vi "input.vi"(8 "error in":errorcluster, 10 "data table in":T1, 11 "dds runtime in":refnum<class "DDS runtime.lvclass">) -> (0 "error out":errorcluster, 2 "data table out":T1, 3 "dds runtime out":refnum<class "DDS runtime.lvclass">)   [LabVIEW 2013, in "DDS runtime.lvclass"]
doc: "Provides an interface for reading data from a module at runtime. While this interface performs no operations, a child should provide an override which may read from any open sessions, references, or interfaces."
uses:
  DDS runtime.lvclass
  <vilib>/NI/Tag Bus/table/data table.ctl
  DDS runtime.lvclass/DDS runtime.ctl
  <vilib>/NI/Tag Bus/table/data polymorphs/write one/write Double.vi
  <vilib>/NI/Tag Bus/table/data polymorphs/write one/write Single.vi
  <vilib>/NI/Tag Bus/table/data polymorphs/write one/write I64.vi
  <vilib>/NI/Tag Bus/table/data polymorphs/write one/write I32.vi
  <vilib>/NI/Tag Bus/table/data polymorphs/write one/write I16.vi
  <vilib>/NI/Tag Bus/table/data polymorphs/write one/write I8.vi
  <vilib>/NI/Tag Bus/table/data polymorphs/write one/write U64.vi
  <vilib>/NI/Tag Bus/table/data polymorphs/write one/write U32.vi
  <vilib>/NI/Tag Bus/table/data polymorphs/write one/write U16.vi
  <vilib>/NI/Tag Bus/table/data polymorphs/write one/write U8.vi
  <vilib>/NI/Tag Bus/table/data polymorphs/write one/write Boolean.vi
  <vilib>/NI/Tag Bus/table/data polymorphs/write one/write String.vi
  <vilib>/RTI DDS Toolkit for LabVIEW/VIs/Read_Num.vi
  <vilib>/RTI DDS Toolkit for LabVIEW/VIs/Read_NumSgl.vi
  <vilib>/RTI DDS Toolkit for LabVIEW/VIs/Read_NumI64.vi
  <vilib>/RTI DDS Toolkit for LabVIEW/VIs/Read_NumI32.vi
  <vilib>/RTI DDS Toolkit for LabVIEW/VIs/Read_NumI16.vi
  <vilib>/RTI DDS Toolkit for LabVIEW/VIs/Read_NumI8.vi
  <vilib>/RTI DDS Toolkit for LabVIEW/VIs/Read_NumU64.vi
  <vilib>/RTI DDS Toolkit for LabVIEW/VIs/Read_NumU32.vi
  <vilib>/RTI DDS Toolkit for LabVIEW/VIs/Read_NumU16.vi
  <vilib>/RTI DDS Toolkit for LabVIEW/VIs/Read_NumU8.vi
  <vilib>/RTI DDS Toolkit for LabVIEW/VIs/Read_Bool.vi
  <vilib>/RTI DDS Toolkit for LabVIEW/VIs/Read_String.vi
  <vilib>/NI/Tag Bus/table/data table.lvlib
  <vilib>/RTI DDS Toolkit for LabVIEW/Library/LVDDS_library.lvlib
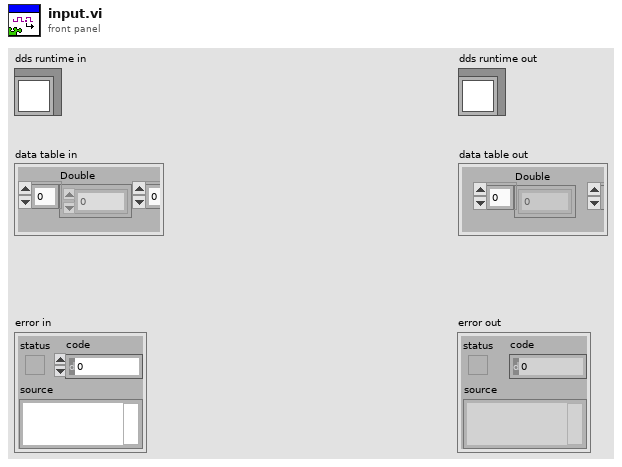
[diagram p1: front panel]
types:
  T1 = typedef "tag bus.lvlib/data table.lvlib/data table.ctl" = cluster{"Double":dbl[], "Single":sgl[], "I64":i64[], "I32":i32[], "I16":i16[], "I8":i8[], "U64":u64[], "U32":u32[], "U16":u16[], "U8":u8[], "Boolean":bool[], "String":string[], "Array of Double":cluster{"DBL Array":dbl[]}[], "Array of Single":cluster{"SGL Array":sgl[]}[], "Array of I64":cluster{"I64 Array":i64[]}[], "Array of I32":cluster{"I32 Array":i32[]}[], "Array of I16":cluster{"I16 Array":i16[]}[], "Array of I8":cluster{"I8 Array":i8[]}[], "Array of U64":cluster{"U64 Array":u64[]}[], "Array of U32":cluster{"U32 Array":u32[]}[], "Array of U16":cluster{"U16 Array":u16[]}[], "Array of U8":cluster{"U8 Array":u8[]}[], "Array of Boolean":cluster{"Boolean Array":bool[]}[], "Array of String":cluster{"String Array":string[]}[]}
  T2 = typedef "tag bus.lvlib/tag descriptor.lvclass/Data Type.ctl" = enum16{"Double", "Single", "I64", "I32", "I16", "I8", "U64", "U32", "U16", "U8", "Boolean", "String", "Array of Double", "Array of Single", "Array of I64", "Array of I32", "Array of I16", "Array of I8", "Array of U64", "Array of U32", "Array of U16", "Array of U8", "Array of Boolean", "Array of String"}
  T3 = cluster{"index":i32, "data type":T2, "ref num":u64, "new samples only":bool, "query condition":string}[]
  T4 = typedef "LVDDS_library.lvlib/DDS Sample Info.ctl" = cluster{"DDS_SampleStateKind":enum32{"DDS_INVALID_SAMPLE_STATE", "DDS_READ_SAMPLE_STATE", "DDS_NOT_READ_SAMPLE_STATE"}, "DDS_ViewStateKind":enum32{"DDS_INVALID_SAMPLE_STATE", "DDS_NEW_VIEW_STATE", "DDS_NOT_NEW_VIEW_STATE"}, "DDS_InstanceStateKind":enum32{"DDS_INVALID_STATE", "DDS_ALIVE_INSTANCE_STATE", "DDS_NOT_ALIVE_DISPOSED_INSTANCE_STATE", "", "DDS_NOT_ALIVE_NO_WRITERS_INSTANCE_STATE"}, "sec":i32, "nanosec":u32, "valid_data":bool}
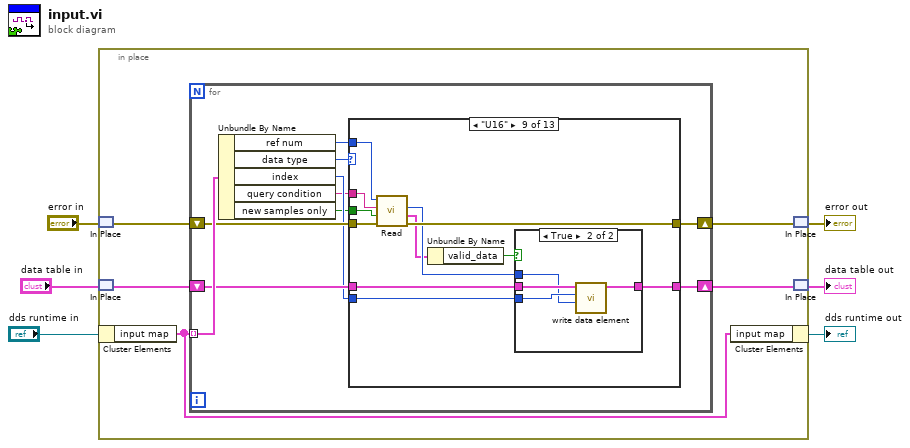
[diagram p0: block diagram]
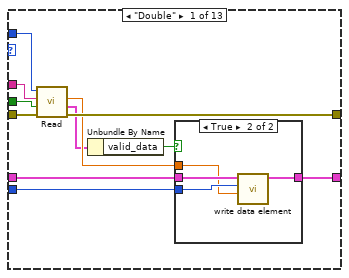
[diagram p2: hidden frame]
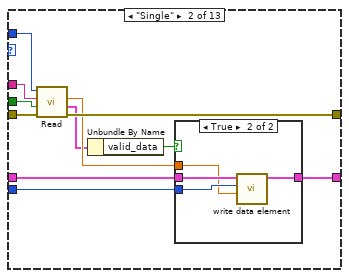
[diagram p4: hidden frame]
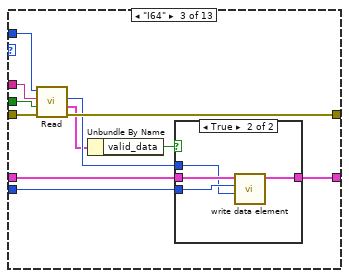
[diagram p6: hidden frame]
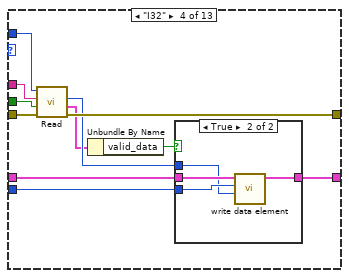
[diagram p8: hidden frame]
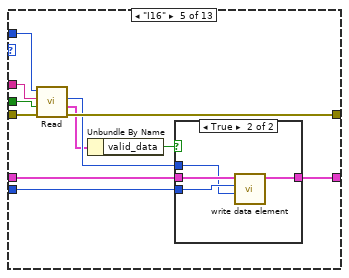
[diagram p10: hidden frame]
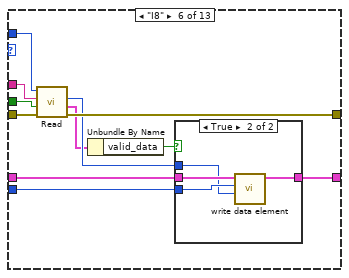
[diagram p12: hidden frame]
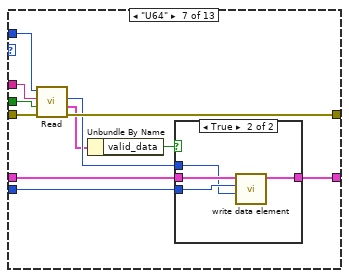
[diagram p14: hidden frame]
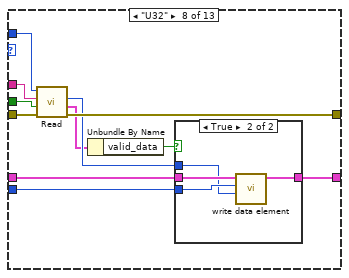
[diagram p16: hidden frame]
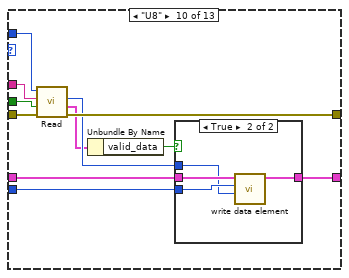
[diagram p19: hidden frame]
diagram:
  n1 = in-place {
    n2 = in-place-match #1("error in") -> (w10:errorcluster)
    n3 = in-place-match #2("data table in") -> (w11:T1)
    n4 = in-place-cluster #3("dds runtime in") -> ("input map"=w7:T3)
    n5 = for {
      tunnel: w7 -> [w21] mode=indexing
      shift-right: [w17] -> w8
      shift-left: w11 -> [w20]
      shift-right: [w18] -> w9
      shift-left: w10 -> [w19]
      n6 = Unbundle By Name(w21) -> ("ref num"=w15:u64, "data type"=w16:T2, "index"=w14:i32, "query condition"=w13:string, "new samples only"=w12:bool)
      n7 = case shown="\"U16\"" w16 {
        tunnel: w20 -> [w29 w45 w61 w77 w93 w109 w125 w141 w157 w173 w189 w205 w215]
        tunnel: w15 -> [w32 w48 w64 w80 w96 w112 w128 w144 w160 w176 w192 w208 _]
        tunnel: w19 -> [w31 w47 w63 w79 w95 w111 w127 w143 w159 w175 w191 w207 w214]
        tunnel: [w30 w46 w62 w78 w94 w110 w126 w142 w158 w174 w190 w206 w214] -> w18
        tunnel: w14 -> [w28 w44 w60 w76 w92 w108 w124 w140 w156 w172 w188 w204 _]
        tunnel: [w26 w42 w58 w74 w90 w106 w122 w138 w154 w170 w186 w202 w215] -> w17
        tunnel: w13 -> [w23 w39 w55 w71 w87 w103 w119 w135 w151 w167 w183 w199 _]
        tunnel: w12 -> [w22 w38 w54 w70 w86 w102 w118 w134 w150 w166 w182 w198 _]
        frame "Double" {
          n8 = call-poly <vilib>:"Read.vi"("error in (no error)"=w31, "only_new_samples"=w22, "query condition"=w23, "ref num in"=w32) -> ("error out"=w30:errorcluster, "dds sample info"=w25:T4, "data"=w27:dbl)  [unwired: 4 in, 1 out]
          n9 = Unbundle By Name(w25) -> ("valid_data"=w24:bool)
          n10 = case shown="True" w24 {
            tunnel: w29 -> [w33 w37]
            tunnel: w28 -> [_ w35]
            tunnel: w27 -> [_ w34]
            tunnel: [w33 w36] -> w26
            frame False {
            }
            frame True {
              n11 = call-poly <vilib>:"write data element.vi"("value"=w34, "index"=w35, "data table in"=w37) -> ("data table out"=w36:T1)  [unwired: 8 in]
            }
          }
        }
        frame "Single" {
          n12 = call-poly <vilib>:"Read.vi"("error in (no error)"=w47, "only_new_samples"=w38, "query condition"=w39, "ref num in"=w48) -> ("error out"=w46:errorcluster, "dds sample info"=w41:T4, "data"=w43:sgl)  [unwired: 4 in, 1 out]
          n13 = Unbundle By Name(w41) -> ("valid_data"=w40:bool)
          n14 = case shown="True" w40 {
            tunnel: w45 -> [w49 w53]
            tunnel: w44 -> [_ w51]
            tunnel: w43 -> [_ w50]
            tunnel: [w49 w52] -> w42
            frame False {
            }
            frame True {
              n15 = call-poly <vilib>:"write data element.vi"("value"=w50, "index"=w51, "data table in"=w53) -> ("data table out"=w52:T1)  [unwired: 8 in]
            }
          }
        }
        frame "I64" {
          n16 = call-poly <vilib>:"Read.vi"("error in (no error)"=w63, "only_new_samples"=w54, "query condition"=w55, "ref num in"=w64) -> ("error out"=w62:errorcluster, "dds sample info"=w57:T4, "data"=w59:i64)  [unwired: 4 in, 1 out]
          n17 = Unbundle By Name(w57) -> ("valid_data"=w56:bool)
          n18 = case shown="True" w56 {
            tunnel: w61 -> [w65 w68]
            tunnel: w60 -> [_ w67]
            tunnel: w59 -> [_ w66]
            tunnel: [w65 w69] -> w58
            frame False {
            }
            frame True {
              n19 = call-poly <vilib>:"write data element.vi"("value"=w66, "index"=w67, "data table in"=w68) -> ("data table out"=w69:T1)  [unwired: 8 in]
            }
          }
        }
        frame "I32" {
          n20 = call-poly <vilib>:"Read.vi"("error in (no error)"=w79, "only_new_samples"=w70, "query condition"=w71, "ref num in"=w80) -> ("error out"=w78:errorcluster, "dds sample info"=w73:T4, "data"=w75:i32)  [unwired: 4 in, 1 out]
          n21 = Unbundle By Name(w73) -> ("valid_data"=w72:bool)
          n22 = case shown="True" w72 {
            tunnel: w77 -> [w81 w84]
            tunnel: w76 -> [_ w83]
            tunnel: w75 -> [_ w82]
            tunnel: [w81 w85] -> w74
            frame False {
            }
            frame True {
              n23 = call-poly <vilib>:"write data element.vi"("value"=w82, "index"=w83, "data table in"=w84) -> ("data table out"=w85:T1)  [unwired: 8 in]
            }
          }
        }
        frame "I16" {
          n24 = call-poly <vilib>:"Read.vi"("error in (no error)"=w95, "only_new_samples"=w86, "query condition"=w87, "ref num in"=w96) -> ("error out"=w94:errorcluster, "dds sample info"=w89:T4, "data"=w91:i16)  [unwired: 4 in, 1 out]
          n25 = Unbundle By Name(w89) -> ("valid_data"=w88:bool)
          n26 = case shown="True" w88 {
            tunnel: w93 -> [w97 w101]
            tunnel: w92 -> [_ w99]
            tunnel: w91 -> [_ w98]
            tunnel: [w97 w100] -> w90
            frame False {
            }
            frame True {
              n27 = call-poly <vilib>:"write data element.vi"("value"=w98, "index"=w99, "data table in"=w101) -> ("data table out"=w100:T1)  [unwired: 8 in]
            }
          }
        }
        frame "I8" {
          n28 = call-poly <vilib>:"Read.vi"("error in (no error)"=w111, "only_new_samples"=w102, "query condition"=w103, "ref num in"=w112) -> ("error out"=w110:errorcluster, "dds sample info"=w105:T4, "data"=w107:i8)  [unwired: 4 in, 1 out]
          n29 = Unbundle By Name(w105) -> ("valid_data"=w104:bool)
          n30 = case shown="True" w104 {
            tunnel: w109 -> [w113 w116]
            tunnel: w108 -> [_ w115]
            tunnel: w107 -> [_ w114]
            tunnel: [w113 w117] -> w106
            frame False {
            }
            frame True {
              n31 = call-poly <vilib>:"write data element.vi"("value"=w114, "index"=w115, "data table in"=w116) -> ("data table out"=w117:T1)  [unwired: 8 in]
            }
          }
        }
        frame "U64" {
          n32 = call-poly <vilib>:"Read.vi"("error in (no error)"=w127, "only_new_samples"=w118, "query condition"=w119, "ref num in"=w128) -> ("error out"=w126:errorcluster, "dds sample info"=w121:T4, "data"=w123:u64)  [unwired: 4 in, 1 out]
          n33 = Unbundle By Name(w121) -> ("valid_data"=w120:bool)
          n34 = case shown="True" w120 {
            tunnel: w125 -> [w129 w132]
            tunnel: w124 -> [_ w131]
            tunnel: w123 -> [_ w130]
            tunnel: [w129 w133] -> w122
            frame False {
            }
            frame True {
              n35 = call-poly <vilib>:"write data element.vi"("value"=w130, "index"=w131, "data table in"=w132) -> ("data table out"=w133:T1)  [unwired: 8 in]
            }
          }
        }
        frame "U32" {
          n36 = call-poly <vilib>:"Read.vi"("error in (no error)"=w143, "only_new_samples"=w134, "query condition"=w135, "ref num in"=w144) -> ("error out"=w142:errorcluster, "dds sample info"=w137:T4, "data"=w139:u32)  [unwired: 4 in, 1 out]
          n37 = Unbundle By Name(w137) -> ("valid_data"=w136:bool)
          n38 = case shown="True" w136 {
            tunnel: w141 -> [w145 w148]
            tunnel: w140 -> [_ w147]
            tunnel: w139 -> [_ w146]
            tunnel: [w145 w149] -> w138
            frame False {
            }
            frame True {
              n39 = call-poly <vilib>:"write data element.vi"("value"=w146, "index"=w147, "data table in"=w148) -> ("data table out"=w149:T1)  [unwired: 8 in]
            }
          }
        }
        frame "U16" {
          n40 = call-poly <vilib>:"Read.vi"("error in (no error)"=w159, "only_new_samples"=w150, "query condition"=w151, "ref num in"=w160) -> ("error out"=w158:errorcluster, "dds sample info"=w153:T4, "Data"=w155:u16)  [unwired: 4 in, 1 out]
          n41 = Unbundle By Name(w153) -> ("valid_data"=w152:bool)
          n42 = case shown="True" w152 {
            tunnel: w157 -> [w161 w164]
            tunnel: w156 -> [_ w163]
            tunnel: w155 -> [_ w162]
            tunnel: [w161 w165] -> w154
            frame False {
            }
            frame True {
              n43 = call-poly <vilib>:"write data element.vi"("value"=w162, "index"=w163, "data table in"=w164) -> ("data table out"=w165:T1)  [unwired: 8 in]
            }
          }
        }
        frame "U8" {
          n44 = call-poly <vilib>:"Read.vi"("error in (no error)"=w175, "only_new_samples"=w166, "query condition"=w167, "ref num in"=w176) -> ("error out"=w174:errorcluster, "dds sample info"=w169:T4, "data"=w171:u8)  [unwired: 4 in, 1 out]
          n45 = Unbundle By Name(w169) -> ("valid_data"=w168:bool)
          n46 = case shown="True" w168 {
            tunnel: w173 -> [w177 w180]
            tunnel: w172 -> [_ w179]
            tunnel: w171 -> [_ w178]
            tunnel: [w177 w181] -> w170
            frame False {
            }
            frame True {
              n47 = call-poly <vilib>:"write data element.vi"("value"=w178, "index"=w179, "data table in"=w180) -> ("data table out"=w181:T1)  [unwired: 8 in]
            }
          }
        }
        frame "Boolean" {
          n48 = call-poly <vilib>:"Read.vi"("error in (no error)"=w191, "only_new_samples"=w182, "query condition"=w183, "ref num in"=w192) -> ("error out"=w190:errorcluster, "dds sample info"=w185:T4, "data"=w187:bool)  [unwired: 4 in, 1 out]
          n49 = Unbundle By Name(w185) -> ("valid_data"=w184:bool)
          n50 = case shown="True" w184 {
            tunnel: w189 -> [w193 w196]
            tunnel: w188 -> [_ w195]
            tunnel: w187 -> [_ w194]
            tunnel: [w193 w197] -> w186
            frame False {
            }
            frame True {
              n51 = call-poly <vilib>:"write data element.vi"("value"=w194, "index"=w195, "data table in"=w196) -> ("data table out"=w197:T1)  [unwired: 8 in]
            }
          }
        }
        frame "String" {
          n52 = call-poly <vilib>:"Read.vi"("error in (no error)"=w207, "only_new_samples"=w198, "query condition"=w199, "ref num in"=w208) -> ("error out"=w206:errorcluster, "dds sample info"=w201:T4, "data"=w203:string)  [unwired: 4 in, 1 out]
          n53 = Unbundle By Name(w201) -> ("valid_data"=w200:bool)
          n54 = case shown="True" w200 {
            tunnel: w205 -> [w209 w213]
            tunnel: w204 -> [_ w211]
            tunnel: w203 -> [_ w210]
            tunnel: [w209 w212] -> w202
            frame False {
            }
            frame True {
              n55 = call-poly <vilib>:"write data element.vi"("value"=w210, "index"=w211, "data table in"=w213) -> ("data table out"=w212:T1)  [unwired: 8 in]
            }
          }
        }
        frame Default {
          # "#TODO\nThis case should never be reached.\nThrow error."
        }
      }
    }
    n56 = in-place-cluster #3("input map"=w7) -> (→"dds runtime out":refnum<class "DDS runtime.lvclass">)
    n57 = in-place-match #1(w9) -> (→"error out":errorcluster)
    n58 = in-place-match #2(w8) -> (→"data table out":T1)
  }
